vi "EnableMallocTraceLinux.vi"() -> ()   [LabVIEW 2013]
uses:
  <vilib>/WebDAVClient/Advanced/Put File.vi
  <vilib>/zip/NI_Unzip.lvlib
  <vilib>/WebDAVClient/NI_WebDAV.lvlib
panel:
  out "error out":errorcluster
  in  "password":string
  in  "username":string="admin"
  in  "Target Architecture":enum16{"x64", "ARM"}(ring)
  # "On Linux RT targets, you can use this VI to enable the 1A test to detect memory\nallocations.  First set the IP address of your target in the project and select the\nappropriate CPU architecture of your target (and password if you have one set).\nThen run this VI, open your 1A test (non-Interval version only) and switch to the\nMalloc Detection tab for more instructions.\nNote: after enabling malloc detection mode with this VI, the 1A test is not meant\nto be used for jitter measurement.  To disable this mode, open the target project\nitem's properties and set the DET_MALLOC Conditional Disable Symbol to False."
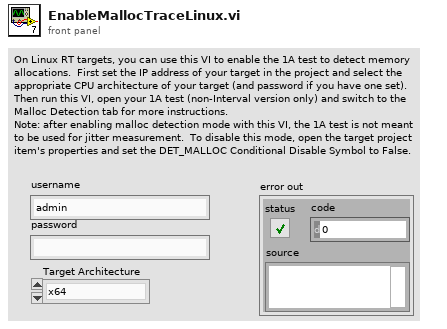
[diagram p1: front panel]
types:
  T1 = typedef "NI_WebDAV.lvlib/SessionHandle.ctl" = refnum<k1>
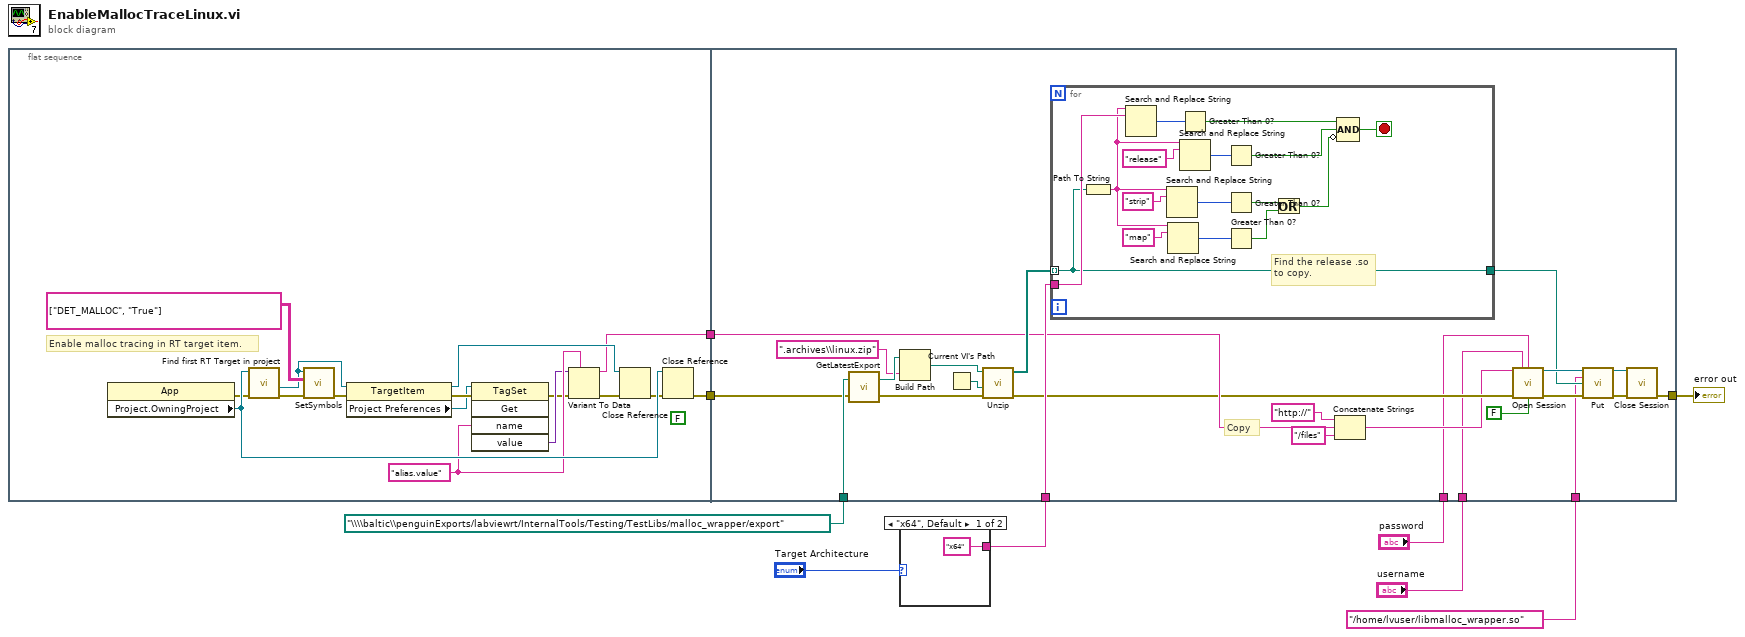
[diagram p0: block diagram]
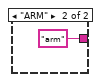
[diagram p2: hidden frame]
diagram:
  n1 = flat-sequence {
    tunnel: [w20] -> w8
    tunnel: [w10] -> w3
    tunnel: path "\\\\baltic\\penguinExports/labviewrt/InternalTools/Testing/TestLibs/malloc_wrapper/export" ("Zip file") -> [w49]
    tunnel: w8 -> [w48]
    tunnel: w6 -> [w42]
    tunnel: "username" -> [w32]
    tunnel: "password" -> [w31]
    tunnel: w3 -> [w39]
    tunnel: "/home/lvuser/libmalloc_wrapper.so" ("string") -> [w34]
    tunnel: [w27] -> w1
    frame #0 {
      (unwired) FALSE ("Is Persistent")
      w14 = "alias.value" ("Name")
      # "Enable malloc tracing in RT target item."
      n2 = property class="App"() -> (error out=w21:errorcluster, "Project.OwningProject"=w24:refnum<vi>)  [unwired: 2 in, 1 out]
      n3 = call "Find first RT Target in project.vi"("error in"=w21, "Project Refnum"=w24) -> ("error out"=w22:errorcluster, "Target"=w16:refnum<vi>)  [unwired: 6 in, 2 out]
      n4 = call <resource>:"SetSymbols.vi"("error in"=w22, "Symbol Value Pairs"=string[][] [["DET_MALLOC", "True"]], "Project Item"=w16) -> ("error out"=w15:errorcluster)  [unwired: 7 in, 1 out]
      n5 = property class="TargetItem"(reference=w16, error in=w15) -> (reference out=w18:refnum<vi>, error out=w19:errorcluster, "Project Preferences"=w17:refnum<vi>)
      n6 = invoke class="TagSet" method="Get"(reference=w17, error in=w19, "name"=w14) -> (error out=w12:errorcluster, "value"=w13:variant)  [unwired: 2 in, 3 out]
      n7 = Variant To Data(error in=w12, type=w14, Variant=w13) -> (data=w10:string, error out=w11:errorcluster)
      n8 = Close Reference(reference=w18, error in (no error)=w11) -> (error out=w23:errorcluster)
      n9 = Close Reference(reference=w24, error in (no error)=w23) -> (error out=w20:errorcluster)
    }
    frame #1 {
      # "Copy"
      n10 = call "GetLatestExport.vi"("error in"=w48, "Export Root"=w49) -> ("error out"=w47:errorcluster, "Latest Root"=w46:path)
      n11 = Build Path(base path=w46, name or relative path=".archives\\linux.zip") -> (appended path=w44:path)
      n12 = Current VI's Path() -> (path=w43:path)
      n13 = call <vilib>:"Unzip.vi"("error in (no error)"=w47, "Target directory (same as Zip file if empty)"=w43, "Zip file"=w44) -> ("error out"=w38:errorcluster, "Unzipped files"=w41:path[])  [unwired: 6 in, 1 out]
      n14 = for {
        tunnel: w42 -> [w65]
        tunnel: w41 -> [w50] mode=indexing
        tunnel: [w50] -> w35
        stop <- w51 stop-if-true
        # "Find the release .so\nto copy."
        n15 = Path To String(path=w50) -> (string=w57:string)
        n16 = Search and Replace String(input string=w57, search string=w65) -> (number of replacements=w64:i32)  [unwired: 6 in, 3 out]
        n17 = Search and Replace String(input string=w57, search string="strip") -> (number of replacements=w60:i32)  [unwired: 6 in, 3 out]
        n18 = Search and Replace String(input string=w57, search string="map") -> (number of replacements=w59:i32)  [unwired: 6 in, 3 out]
        n19 = Greater Than 0?(x=w64) -> (x > 0?=w62:bool)
        n20 = Search and Replace String(input string=w57, search string="release") -> (number of replacements=w63:i32)  [unwired: 6 in, 3 out]
        n21 = Greater Than 0?(x=w63) -> (x > 0?=w61:bool)
        n22 = Greater Than 0?(x=w60) -> (x > 0?=w54:bool)
        n23 = Greater Than 0?(x=w59) -> (x > 0?=w53:bool)
        n24 = Or(x=w54, y=w53) -> (x .or. y?=w52:bool)
        n25 = Compound Arithmetic op=AND(w62, w61, invert w52) -> (w51:bool)
      }
      n26 = Concatenate Strings("http://" ("file uri"), w39, "/files" ("string")) -> (w33:string)
      n27 = call <vilib>:"Open Session.vi"("host uri prefix"=w33, "username"=w32, "password"=w31, "error in (no error)"=w38, "verify server?"=FALSE) -> ("session handle out"=w36:T1, "error out"=w37:errorcluster)  [unwired: 9 in]
      n28 = call-poly <vilib>:"Put.vi"("session handle"=w36, "relative uri"=w34, "local file path"=w35, "error in (no error)"=w37) -> ("session handle out"=w29:T1, "error out"=w28:errorcluster)  [unwired: 9 in, 1 out]
      n29 = call <vilib>:"Close Session.vi"("session handle"=w29, "error in (no error)"=w28) -> ("error out"=w27:errorcluster)  [unwired: 13 in]
    }
  }
  n30 = case shown="\"x64\", Default" "Target Architecture" {
    tunnel: ["x64" ("name or relative path") "arm" ("name or relative path")] -> w6
    frame "x64", Default {
    }
    frame "ARM" {
    }
  }
  "error out" <- w1
